vi "Focus Close.vi"(8 "error in (no error)":errorcluster, 11 "ArduinoFocus in":refnum<class "ArduinoFocus.lvclass">) -> (0 "error out":errorcluster, 3 "ArduinoFocus out":refnum<class "ArduinoFocus.lvclass">)   [LabVIEW 2022 SP3, in "ArduinoFocus.lvclass"]
uses:
  ArduinoFocus.lvclass
  Focus Class/Focus Class.lvclass
  ArduinoFocus.lvclass/ArduinoFocus.ctl
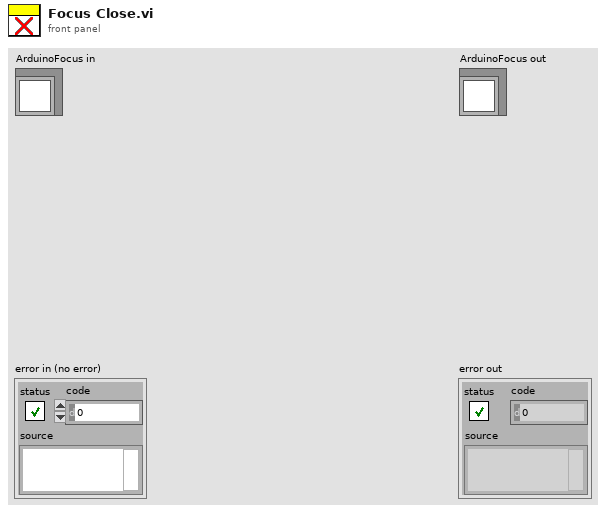
[diagram p1: front panel]
types:
  T1 = typedef "ArduinoFocus.lvclass/Arduino Focus cluster Settings.ctl" = cluster{"Port":refnum<visa-resource-name>, "Homing Parameters":T2, "Positions":i32[], "Homed":bool[]}
  T2 = typedef "arduino Motor Control cluster Command.ctl" = cluster{"Direction":bool, "NUMBER OF  STEPS":u32, "SPEED STEPS/SEC":u16, "ACC/DECEL STEPS/SEC^2":u16, "EN/DIS?":bool}
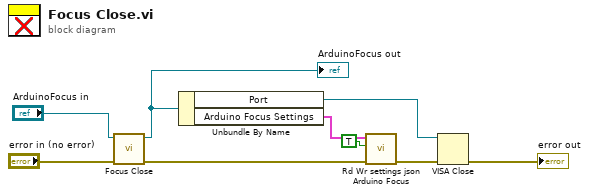
[diagram p0: block diagram]
diagram:
  n1 = call-parent "Focus Close.vi"("error in (no error)"="error in (no error)", "Focus Class in"="ArduinoFocus in") -> ("error out"=w4:errorcluster, "Focus Class out"=w7:refnum<class "ArduinoFocus.lvclass">)  [unwired: 8 in]
  "ArduinoFocus out" <- w7
  n2 = Unbundle By Name(w7) -> ("Port"=w3:refnum<visa-resource-name>, "Arduino Focus Settings"=w6:T1)
  n3 = call "Rd Wr settings json Arduino Focus.vi"("error in (no error)"=w4, "Write? (F:Read)"=TRUE, "Arduino Focus Settings"=w6) -> ("error out"=w2:errorcluster)  [unwired: 7 in, 1 out]
  n4 = VISA Close(VISA resource name=w3, error in (no error)=w2) -> (error out=→"error out":errorcluster)
